vi "(SubVI) Get handle_YCC.vi"(1 "Incoming Handle":i32) -> (0 "Outgoing Handle":i32)   [LabVIEW 2014]
uses:
  MCL-dll-Labview 32-bit/Madlib.dll
panel:
  # "This VI implements an initialization sequence for use with \na single Nano-Drive."
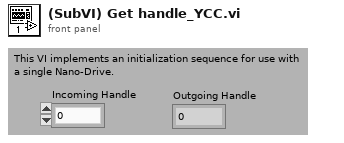
[diagram p1: front panel]
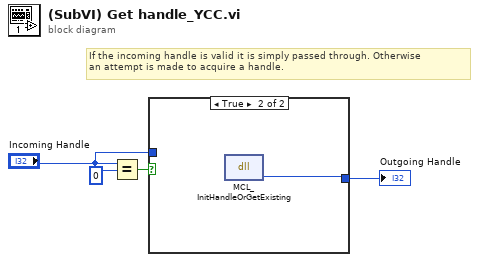
[diagram p0: block diagram]
diagram:
  # "If the incoming handle is valid it is simply passed through. Otherwise\nan attempt is made to acquire a handle."
  n1 = Equal?(x="Incoming Handle", y=0) -> (x = y?=w3:bool)
  n2 = case shown="True" w3 {
    tunnel: [w5 w6] -> w1
    tunnel: "Incoming Handle" -> [w5 _]
    frame False {
    }
    frame True {
      n3 = dll-call lib="C:/Users/hwLi-lab/Desktop/YCC's OT/Main-Stage-Based/SubVI-Stage-Based/MCL-dll-Labview 32-bit/Madlib.dll" fn="MCL_InitHandleOrGetExisting"() -> ("return type"=w6:i32)  [unwired: 3 in, 2 out]
    }
  }
  "Outgoing Handle" <- w1
